vi "Get Project MyComputer.vi"(8 "error in":errorcluster) -> (0 "error out":errorcluster, 3 "My Computer":refnum<vi>)   [LabVIEW 2020, in "Missing in Project.lvclass"]
doc: "Returns the MyComputer reference to the project."
uses:
  Missing in Project.lvclass
panel:
  out "project path":path
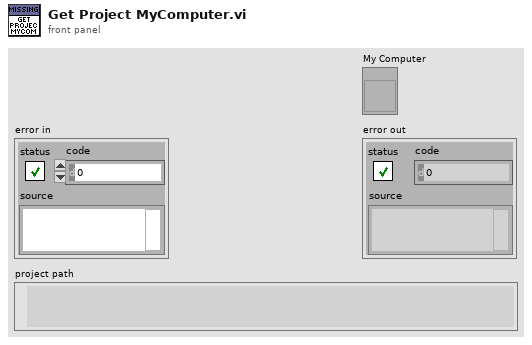
[diagram p1: front panel]
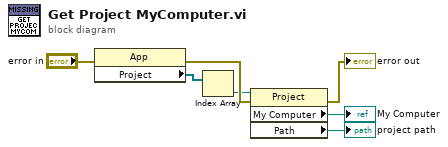
[diagram p0: block diagram]
diagram:
  n1 = property class="App"(error in="error in") -> (error out=w5:errorcluster, "Project"=w3:refnum<vi>[])  [unwired: 1 in, 1 out]
  n2 = Index Array(array=w3) -> (element=w2:refnum<vi>)  [unwired: 1 in]
  n3 = property class="Project"(reference=w2, error in=w5) -> (error out=→"error out":errorcluster, "My Computer"=→"My Computer":refnum<vi>, "Path"=→"project path":path)  [unwired: 1 out]
